vi "HVPPS Class Ref.vi"(6 "Option":T1, 8 "error in":errorcluster, 10 "Socket No":u16, 11 "VT_LTT.lvlib:IT-M6018C.lvclass_In":refnum<class "IT-M6018C.lvclass">) -> (0 "error out":errorcluster, 3 "VT_LTT.lvlib:IT-M6018C.lvclass_out":refnum<class "IT-M6018C.lvclass">)   [LabVIEW 2023, in "HardwareAbstractionLayer_LVOOP.lvlib" / "Wait Monitor.lvclass"]
uses:
  Wait Monitor.lvclass
  Control/PPS FGV Option.ctl
  PowerSupply/IT-M6018C/IT-M6018C.lvclass
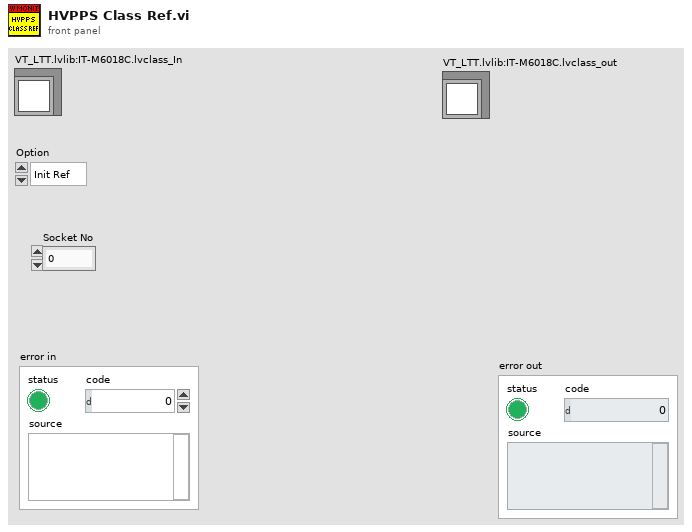
[diagram p1: front panel]
types:
  T1 = typedef "HardwareAbstractionLayer_LVOOP.lvlib/Wait Monitor.lvclass/PPS FGV Option.ctl" = enum16{"Init Ref", "Get Ref", "Set Ref"}
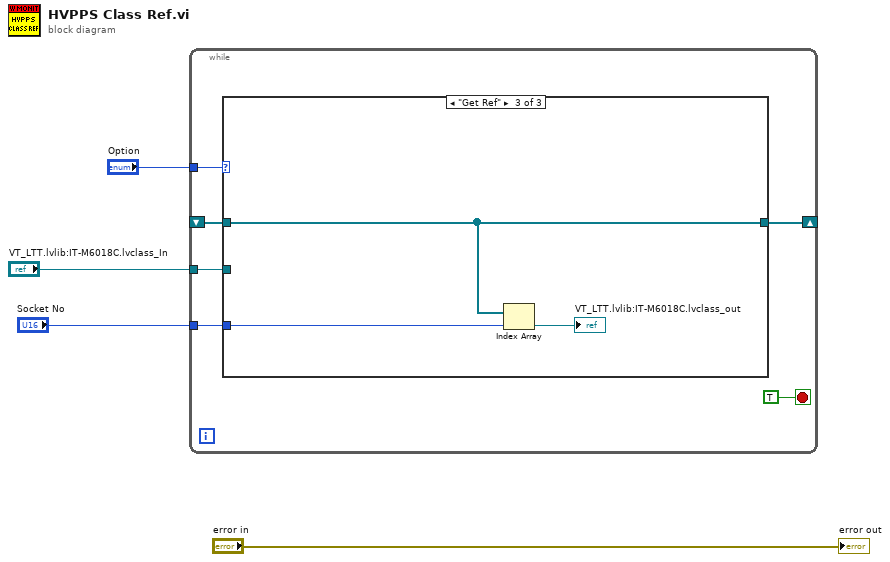
[diagram p0: block diagram]
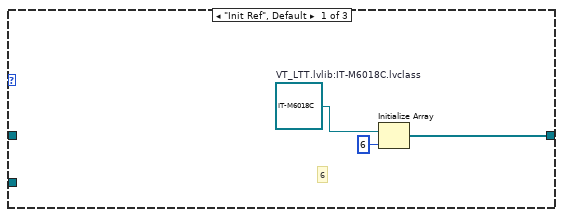
[diagram p2: hidden frame]
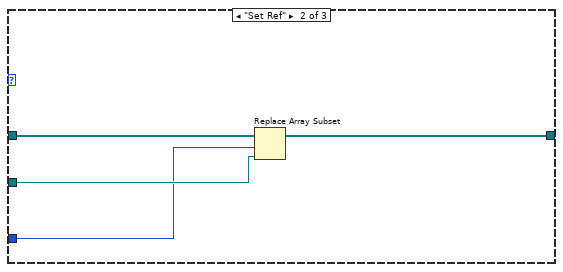
[diagram p3: hidden frame]
diagram:
  n1 = while {
    tunnel: "Option" -> [w9]
    shift-right: [w8] -> _
    shift-left: _ -> [w7]
    tunnel: "VT_LTT.lvlib:IT-M6018C.lvclass_In" -> [w6]
    tunnel: "Socket No" -> [w5]
    stop <- TRUE stop-if-true
    n2 = case shown="\"Get Ref\"" w9 {
      tunnel: [w11 w16 w20] -> w8
      tunnel: w7 -> [_ w17 w20]
      tunnel: w6 -> [_ w15 _]
      tunnel: w5 -> [_ w14 w18]
      frame "Init Ref", Default {
        w13 = refnum<class "IT-M6018C.lvclass"> refnum  # VT_LTT.lvlib:IT-M6018C.lvclass
        # "6"
        n3 = Initialize Array(w13, 6 ("dimension size")) -> (w11:refnum<class "IT-M6018C.lvclass">[])
      }
      frame "Set Ref" {
        n4 = Replace Array Subset(array=w17, new element=w15, index=w14) -> (w16:refnum<class "IT-M6018C.lvclass">[])
      }
      frame "Get Ref" {
        n5 = Index Array(array=w20, index=w18) -> (element=→"VT_LTT.lvlib:IT-M6018C.lvclass_out":refnum<class "IT-M6018C.lvclass">)
      }
    }
  }
  "error out" <- "error in"
